vi "Txt to clean Array (Dashboard).vi"(3 "error in":errorcluster, 4 "Overide":bool, 5 "Variables":string, 6 "file path":path=path "C:/Users/usr/Desktop/FRC/2014 code/Robot Constants 2-3-14.txt") -> (0 "error out":errorcluster, 1 "Variable Names":string[](array[string]), 2 "Array of Numbers":dbl[](array[numeric]))   [LabVIEW 2013]
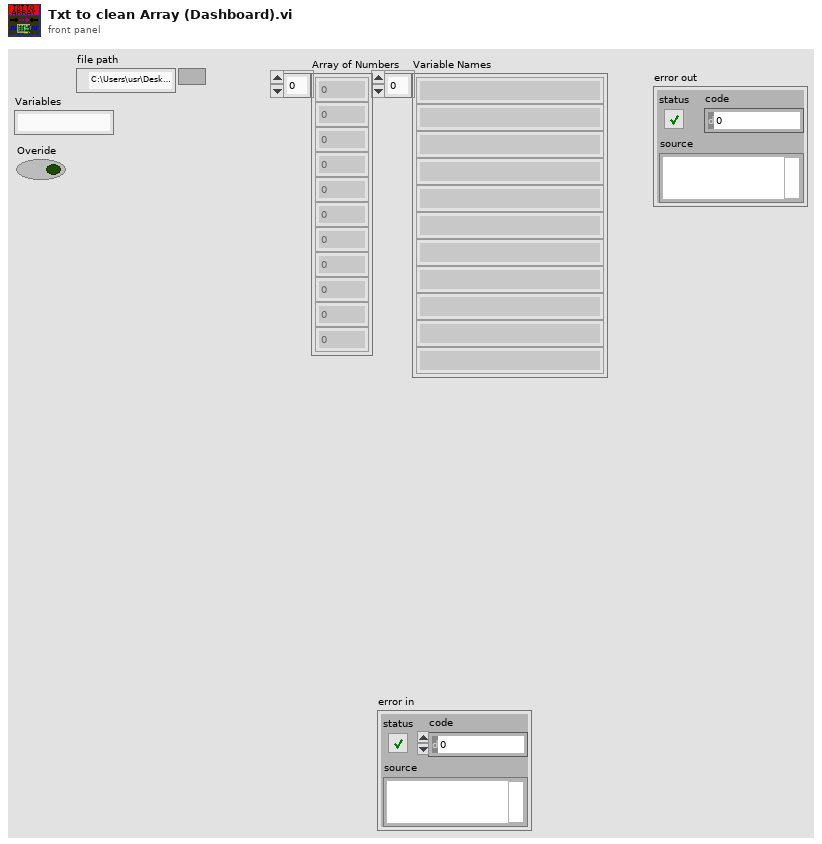
[diagram p1: front panel]
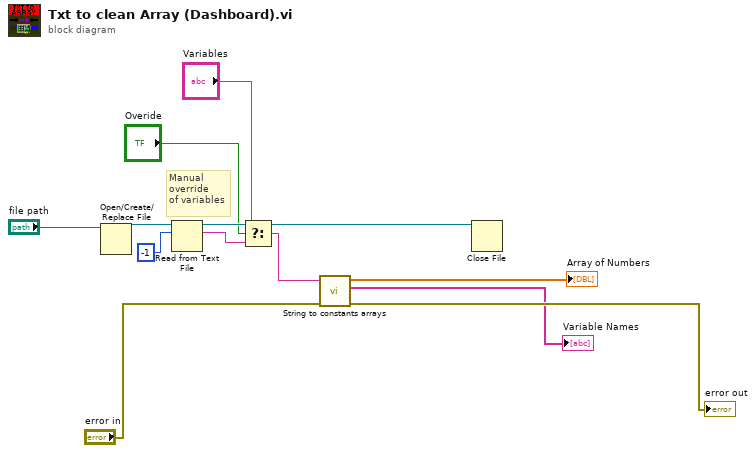
[diagram p0: block diagram]
diagram:
  # "Manual\noverride\nof variables"
  n1 = Open/Create/Replace File(file path (use dialog)="file path") -> (refnum out=w11:refnum<file>)  [unwired: 5 in, 2 out]
  n2 = Read from Text File(file (use dialog)=w11, count=-1) -> (refnum out=w10:refnum<file>, text=w5:string)  [unwired: 2 in, 2 out]
  n3 = Select(t="Variables", s="Overide", f=w5) -> (s? t:f=w6:string)
  n4 = call "String to constants arrays.vi"("error in (no error)"="error in", "Variables"=w6) -> ("error out"=→"error out":errorcluster, "Variable Names"=→"Variable Names":string[], "Array of Numbers"=→"Array of Numbers":dbl[])  [unwired: 7 in]
  n5 = Close File(refnum=w10) -> ()  [unwired: 1 in, 2 out]
